vi "Enqueue ECU Action.vi"(6 "Prioritize Data?":bool, 8 "error in":errorcluster, 10 "Command":variant, 11 "Message":string) -> (0 "error out":errorcluster)   [LabVIEW 2024, in "RT Management.lvlib"]
uses:
  RT Management.lvlib
  ECU Internal Communications/QMH Item.ctl
  ECU Internal Communications/Queues - Get.vi
  ECU Internal Communications/ECU InterComm.lvlib
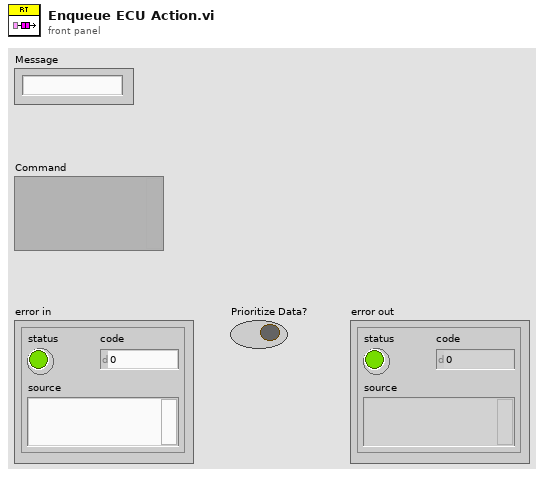
[diagram p1: front panel]
types:
  T1 = typedef "ECU InterComm.lvlib/QMH Item.ctl" = cluster{"Message":string, "Data":variant}
  T2 = typedef "ECU InterComm.lvlib/Process Queues.ctl" = cluster{"Incoming Requests":refnum<queue>, "ECU Working Mode":refnum<queue>}
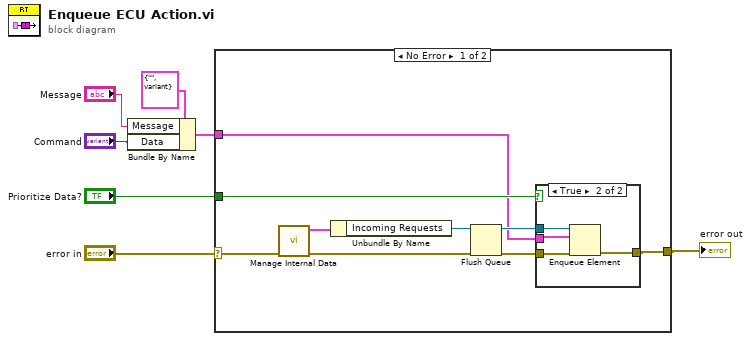
[diagram p0: block diagram]
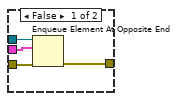
[diagram p2: hidden frame]
diagram:
  n1 = Bundle By Name(cluster=T1 {"Message"="", "Data"=variant} ("Cluster"), "Message"="Message", "Data"="Command") -> (w5:T1)
  n2 = case shown="No Error" "error in" {
    selector: "error in" -> [w14 w25]
    tunnel: "Prioritize Data?" -> [w15 _]
    tunnel: [w13 w25] -> w1
    tunnel: w5 -> [w8 _]
    frame No Error {
      n3 = call-poly "Manage Internal Data.vi"("error in"=w14) -> ("error out"=w12:errorcluster, "Queues Out"=w16:T2)  [unwired: 9 in]
      n4 = Unbundle By Name(w16) -> ("Incoming Requests"=w11:refnum<queue>)
      n5 = Flush Queue(queue=w11, error in (no error)=w12) -> (queue out=w10:refnum<queue>, error out=w9:errorcluster)  [unwired: 1 out]
      n6 = case shown="True" w15 {
        tunnel: w10 -> [w19 w24]
        tunnel: w9 -> [w20 w23]
        tunnel: [w18 w22] -> w13
        tunnel: w8 -> [w17 w21]
        frame False {
          n7 = Enqueue Element At Opposite End(queue=w19, element=w17, error in (no error)=w20) -> (error out=w18:errorcluster)  [unwired: 1 in, 2 out]
        }
        frame True {
          n8 = Enqueue Element(queue=w24, element=w21, error in (no error)=w23) -> (error out=w22:errorcluster)  [unwired: 1 in, 2 out]
        }
      }
    }
    frame Error {
    }
  }
  "error out" <- w1
